vi "Load State Data.vi"(8 "error in (no error)":errorcluster, 11 "PieChart in":refnum<class "PieChart.lvclass">) -> (0 "error out":errorcluster, 3 "PieChart out":refnum<class "PieChart.lvclass">)   [LabVIEW 2020, in "PieChart.lvclass"]
doc: "The <b>Load State Data VI</b> is a dynamic dispatch VI that must be overwritten in every QControl Class that uses the State Data. If used it must <b>Call Parent Method</b>. This recursively loads the Data Value Reference to the data space for the QControl Class up the inheritance hierarchy that uses the Data Value Reference.\n<b> </b> <b> </b>\n©2016 Q Software Innovations, LLC (QSI)\nwritten by Quentin Alldredge\nproduced in LabVIEW 2015\n\nsupport@qsoftwareinnovations.com\nwww.qsoftwareinnovations.com\n\nAll rights reserved.\n\nRedistribution and use in source and binary forms, with or without modification, are permitted provided that the following conditions are met:\n\n * Redistributions of source code must retain the above copyright notice, this list of conditions and the following disclaimer.\n * Redistributions in binary form must reproduce the above copyright notice, this list of conditions and the following disclaimer in the documentation and/or other materials provided with the distribution.\n * Neither the name of Q Software Innovations, LLC. nor the names of its contributors may be used to endorse or promote products derived from this software without specific prior written permission.\n\nTHIS SOFTWARE IS PROVIDED BY THE COPYRIGHT HOLDERS AND CONTRIBUTORS \"AS IS\" AND ANY EXPRESS OR IMPLIED WARRANTIES, INCLUDING, BUT NOT LIMITED TO, THE IMPLIED WARRANTIES OF MERCHANTABILITY AND FITNESS FOR A PARTICULAR PURPOSE ARE DISCLAIMED. IN NO EVENT SHALL THE COPYRIGHT OWNER OR CONTRIBUTORS BE LIABLE FOR ANY DIRECT, INDIRECT, INCIDENTAL, SPECIAL, EXEMPLARY, OR CONSEQUENTIAL DAMAGES (INCLUDING, BUT NOT LIMITED TO, PROCUREMENT OF SUBSTITUTE GOODS OR SERVICES; LOSS OF USE, DATA, OR PROFITS; OR BUSINESS INTERRUPTION) HOWEVER CAUSED AND ON ANY THEORY OF LIABILITY, WHETHER IN CONTRACT, STRICT LIABILITY, OR TORT (INCLUDING NEGLIGENCE OR OTHERWISE) ARISING IN ANY WAY OUT OF THE USE OF THIS SOFTWARE, EVEN IF ADVISED OF THE POSSIBILITY OF SUCH DAMAGE."
uses:
  PieChart.lvclass
  State Data.ctl
  <vilib>/Utility/miscctls.llb/LVFontTypeDef.ctl
  Pie info for Click.ctl
  <vilib>/Utility/miscctls.llb/LVBoundsTypeDef.ctl
  PieChart.lvclass/PieChart.ctl
  <vilib>/QSI/QControls/QControl Classes/Picture/Picture.lvclass
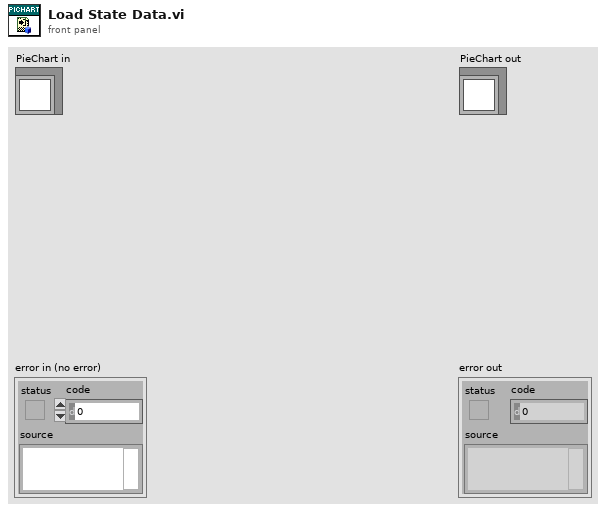
[diagram p1: front panel]
types:
  T1 = typedef "LVFontTypeDef.ctl" = cluster{"Font Name":string, "Size":u16, "Bold":bool, "Italic":bool, "Underline":bool, "Strikeout":bool, "Color":u32}
  T2 = typedef "PieChart.lvclass/State Data.ctl" = cluster{"Title":string, "Values[]":dbl[], "Labels[]":string[], "Colors[]":u32[], "Include Legend?":bool, "Include Title?":bool, "Title Font":T1, "Legend Font":T1, "Selection":i32, "Slice Positions":T3}
  T3 = typedef "PieChart.lvclass/Pie info for Click.ctl" = cluster{"Slice Positions":cluster{"Start":i16, "End":i16}[], "Center Position":T4, "Radius":i16}
  T4 = typedef "LVBoundsTypeDef.ctl" = cluster{"Width":u32, "Height":u32}
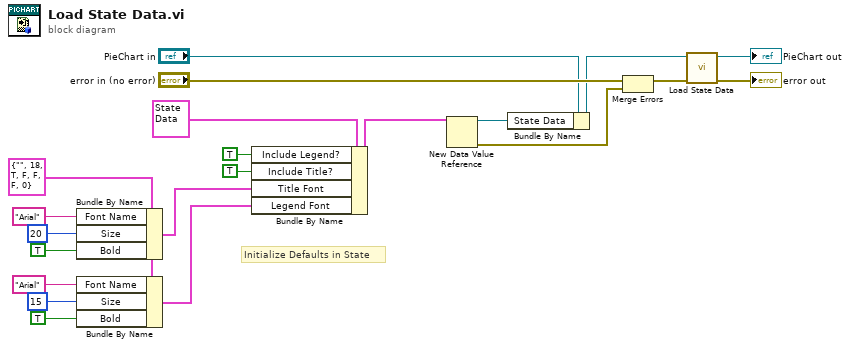
[diagram p0: block diagram]
diagram:
  w2 = T1 {"Font Name"="", "Size"=18, "Bold"=TRUE, "Italic"=FALSE, "Underline"=FALSE, "Strikeout"=FALSE, "Color"=0} ("Title Font")
  # "Initialize Defaults in State"
  n1 = Bundle By Name(cluster=w2, "Font Name"="Arial", "Size"=u16 20, "Bold"=TRUE) -> (w6:T1)
  n2 = Bundle By Name(cluster=w2, "Font Name"="Arial", "Size"=u16 15, "Bold"=TRUE) -> (w1:T1)
  n3 = Bundle By Name(cluster=T2 {"Title"="", "Values[]"=[], "Labels[]"=[], "Colors[]"=[], "Include Legend?"=FALSE, "Include Title?"=FALSE, "Title Font"={"Font Name"="", "Size"=0, "Bold"=FALSE, "Italic"=FALSE, "Underline"=FALSE, "Strikeout"=FALSE, "Color"=0}, "Legend Font"={"Font Name"="", "Size"=0, "Bold"=FALSE, "Italic"=FALSE, "Underline"=FALSE, "Strikeout"=FALSE, "Color"=0}, "Selection"=2, "Slice Positions"={"Slice Positions"=[], "Center Position"={"Width"=0, "Height"=0}, "Radius"=0}} ("State Data"), "Include Legend?"=TRUE, "Include Title?"=TRUE, "Title Font"=w6, "Legend Font"=w1) -> (w12:T2)
  n4 = New Data Value Reference(data value=w12) -> (data value reference=w16:refnum<data-value>, error out=w14:errorcluster)  [unwired: 1 in]
  n5 = Bundle By Name(cluster="PieChart in", "State Data"=w16) -> (w17:refnum<class "PieChart.lvclass">)
  n6 = Merge Errors("error in (no error)", w14) -> (w15:errorcluster)
  n7 = call-parent "Load State Data.vi"("error in (no error)"=w15, "Control in"=w17) -> ("error out"=→"error out":errorcluster, "Control out"=→"PieChart out":refnum<class "PieChart.lvclass">)  [unwired: 8 in]
